vi "Module_p_control_sing_v1.vi"() -> ()   [LabVIEW 2014]
uses:
  <vilib>/rvi/FXPMathLib/FxpAtan2/subVIs/nifxpmath_Atan2_SimConfig.ctl
  <vilib>/rvi/FXPMathLib/FxpSinAndCos/subVIs/nifxpmath_SinAndCos_SimConfig.ctl
  <vilib>/rvi/Emulation/niFpgaGetClockAttributes.vi
  <vilib>/rvi/Emulation/niFpgaSctlEmulationGetInTimedLoop.vi
  <vilib>/rvi/Emulation/niFpgaEmulationReportErrorSimple.vi
  <vilib>/rvi/eio/common/nirviEmuTemplateMethod_errors.vi
  <vilib>/rvi/Emulation/niFpgaProcessEmulError.vi
  <vilib>/rvi/Emulation/niFpgaCriticalErrorInLSC.vi
  <vilib>/rvi/interface/RandomDataEmulation/nirviRandomDataMultiElementFPGAFIFO.vi
  <instcachedir>/0/nirviRandomDataMultiElementFPGAFIFO_AD0CFC12EF974623A9C2E4184BC062B2.lvgen/nirviRandomDataMultiElementFPGAFIFO_AD0CFC12EF974623A9C2E4184BC062B2_023.vi
  <vilib>/rvi/interface/RandomDataEmulation/niFpgaRandomDataHandleErrors.vi
  <vilib>/rvi/FXPMathLib/FxpSinAndCos/simVIs/DllFxpSinAndCosTemp_sub.vi
  <vilib>/rvi/FXPMathLib/FxpAtan2/simVIs/DllFxpAtan2Temp_sub.vi
  <vilib>/eio/EIONode/EIONode.xnode
  <vilib>/rvi/FXPMathLib/FxpMul/XNode/nifxpmath_Multiplier.xnode
  <vilib>/rvi/FXPMathLib/FxpSub/XNode/nifxpmath_Sub.xnode
  <vilib>/rvi/FXPMathLib/FxpAdd/XNode/nifxpmath_Add.xnode
  <vilib>/rvi/Analysis/measure/butterworth/XNode/niFpgaButterworthFilter.xnode
  <vilib>/rvi/DataTransferAndStorage/Container/XNode/niFpgaContainer.xnode
  <vilib>/rvi/interface/RandomDataEmulation/nirviRandomDataFpgaMultiElementTemplate.vi
  <vilib>/rvi/FXPMathLib/FxpSinAndCos/XNode/nifxpmath_SinAndCos.xnode
  <vilib>/rvi/FXPMathLib/FxpAtan2/XNode/nifxpmath_Atan2.xnode
  <vilib>/rvi/FXPMathLib/sim/FxpSim.dll
panel:
  in  "Dy_d_M_avg_Tc (uSec)":u32 caption="M_avg_Tc (uSec)"
  out "Omega_y(rad/s)":fxp<+/-,32,18>
  out "Omega_y(M_avg)":fxp<+/-,32,18>
  out "Omega_y(M)":fxp<+/-,32,18>
  in  "Count(s)":u32
  out "Boolean":bool
  out "Dy_temp":fxp<+/-,22,7>
  in  "Sin ini":bool
  out "Dy_dd":fxp<+/-,25,15>
  in  "scaled coefficients_Dy_dd":i32[](array[numeric])=[1067016412, 3362706]
  in  "Dyr":fxp<+/-,22,8>
  out "Dabr_sin/cos":fxp<+/-,22,8>
  in  "Sin_offset_y":fxp<+/-,12,8>
  in  "Sin_magnitude_y":fxp<+/-,11,8>
  out "Dabr_d":fxp<+/-,33,10>
  out "Sin_omega":fxp<+,29,9>
  out "Dabr_dd":fxp<+/-,34,12>
  in  "Sin wave frenqueny (Hz)":fxp<+,21,5>
  out "Dy_d(M_avg method)":fxp<+/-,32,12>
  in  "Dy_d_M_Tc (mSec)":u32 format="%#_6f"
  out "Dy_d(M method)":fxp<+/-,32,12>
  in  "Method case":i32
  out "Dy_d(T method)":fxp<+/-,32,12>
  in  "mt0_omega":u32
  out "mt_omega":u32
  out "Dy_d(mm/s)":fxp<+/-,32,12>
  out "Sin wave time (s)":fxp<+,64,32>
  in  "Coe Ini":bool
  in  "Encoder Reset_y":bool
  in  "Stop Motor_y":bool
  in  "Kd_y":fxp<+,26,2>
  in  "Kp_y":fxp<+,11,7>=0.375
  out "Dy_error":fxp<+/-,21,11>
  out "Dy_PID":fxp<+/-,21,11>
  in  "Dy_tolerance":fxp<+,32,9>=1.0
  out "Encoder Position_y":i32
  out "rad(NrTheta)_y":fxp<+/-,33,18> format="%.21g"
  out "Dy(mm)":fxp<+/-,22,7>
  out "Omega_y(T)":fxp<+/-,20,9>
  out "vq_y_F":fxp<+/-,20,5> format="%.57g"
  out "vd_y_F":fxp<+/-,20,5>
  out "va_y":fxp<+/-,20,5> format="%.21g"
  out "vb_y":fxp<+/-,20,5> format="%.21g"
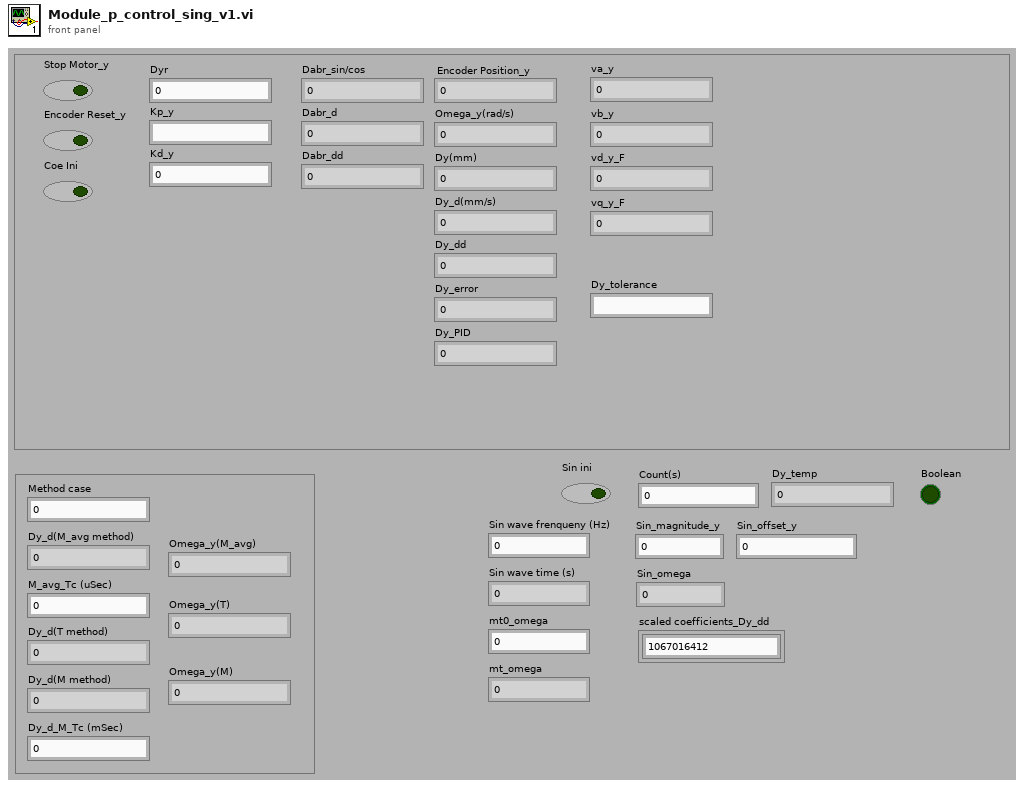
[diagram p1: front panel]
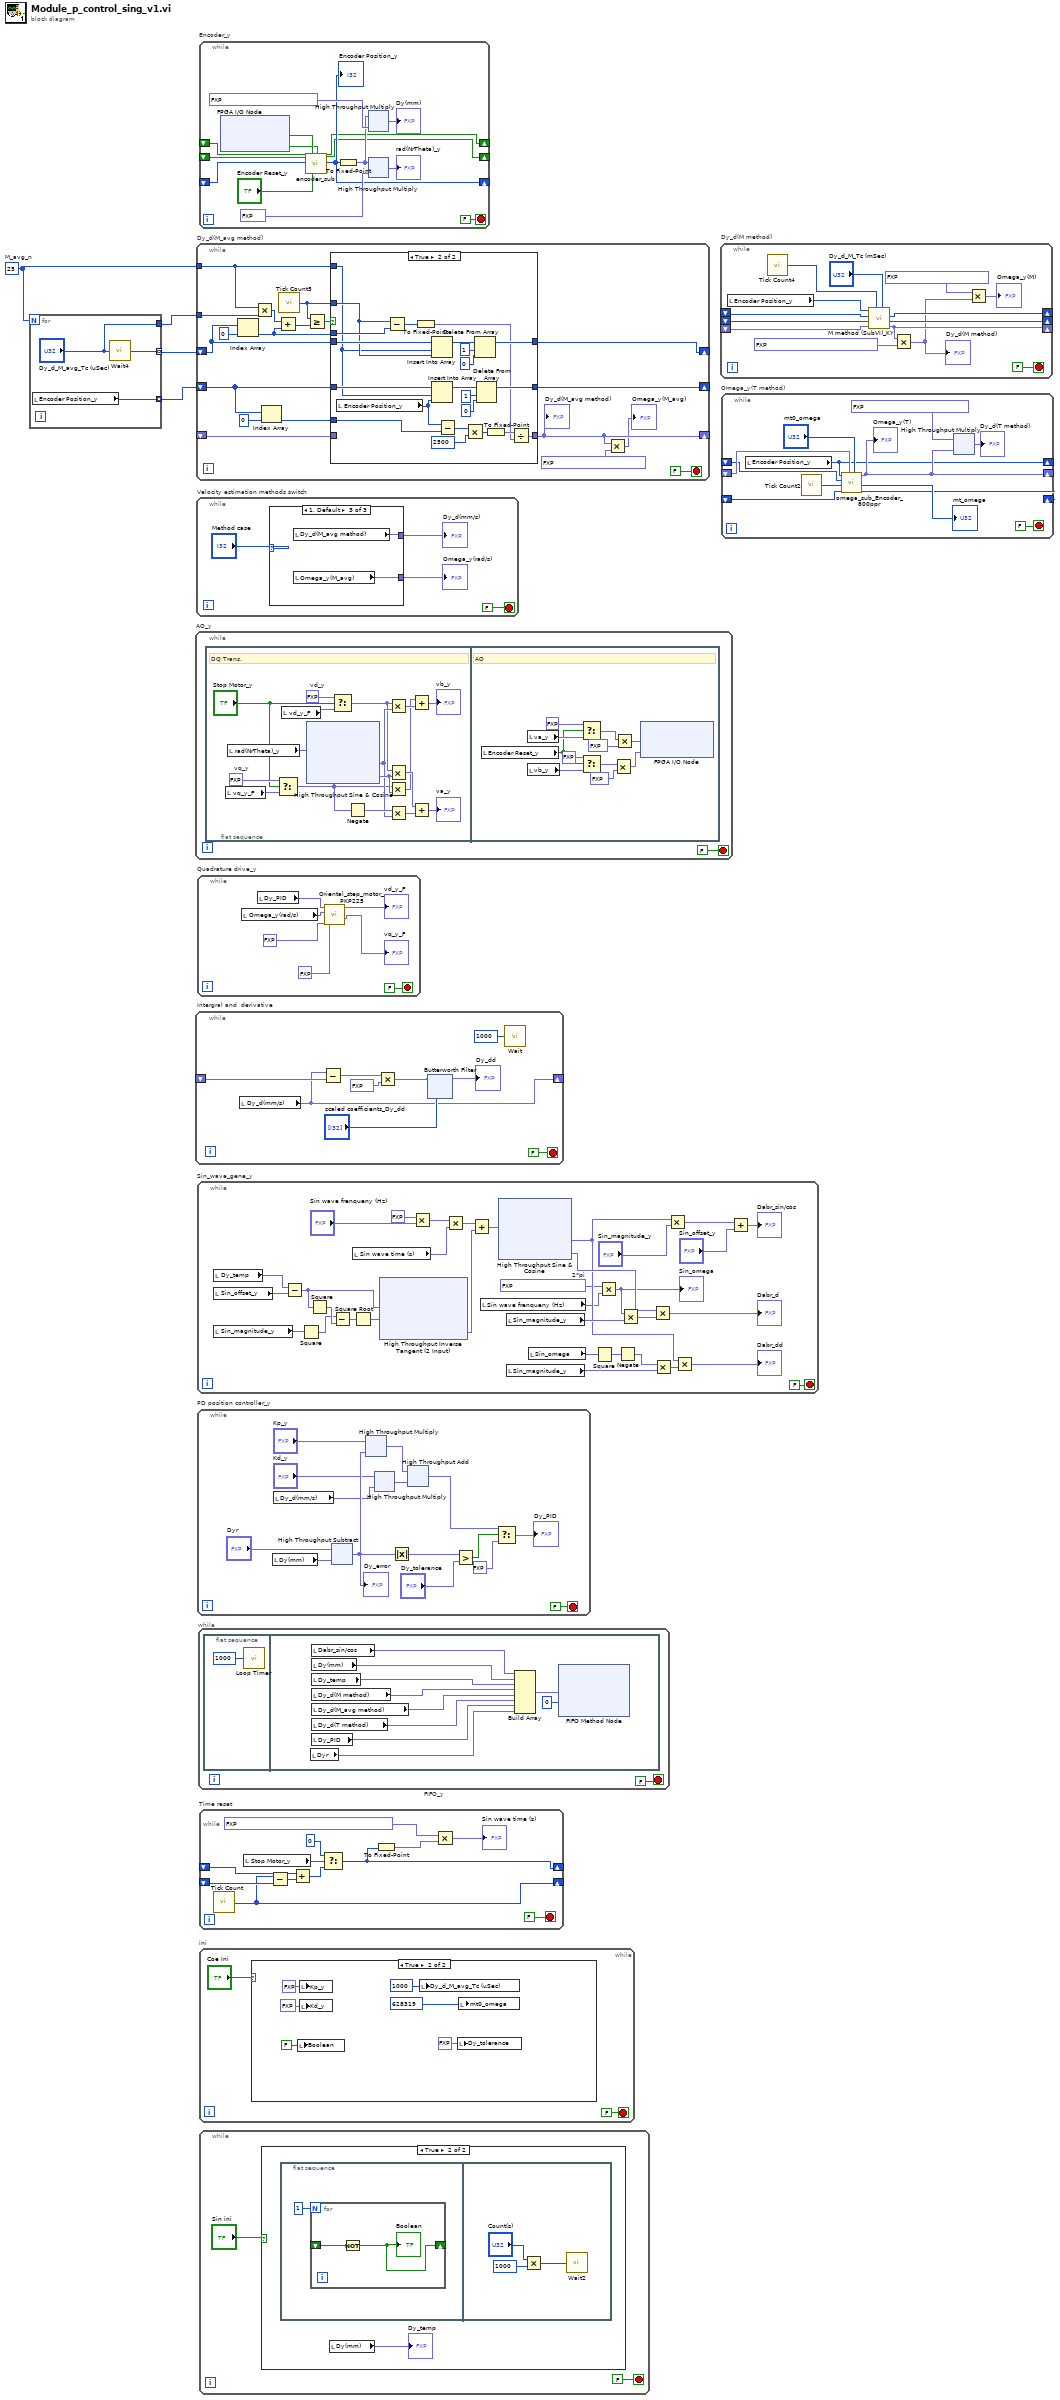
[diagram p0: block diagram]
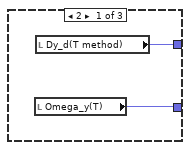
[diagram p4: hidden frame]
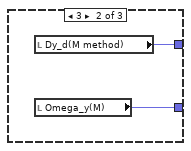
[diagram p5: hidden frame]
diagram:
  w3 = 25  # M_avg_n
  n1 = for {
    N: w3 -> [_]
    tunnel: [w7] -> w1 mode=indexing
    tunnel: [w5] -> w2 mode=indexing
    tunnel: ["Dy_d_M_avg_Tc (uSec)"] -> w4
    n2 = local read "Encoder Position_y"() -> (w5:i32)
    n3 = call "Wait4"("Count(uSec)"="Dy_d_M_avg_Tc (uSec)") -> ("Tick Count(uSec)"=w7:u32)
  }
  n4 = while "AO_y" {
    stop <- FALSE stop-if-true
    n5 = flat-sequence {
      frame #0 {
        w15 = fxp<+/-,20,5> 0.0  # vq_y
        w14 = fxp<+/-,20,5> 0.0  # vd_y
        # "DQ Trans."
        n6 = local read "vq_y_F"() -> (w12:fxp<+/-,20,5>)
        n7 = local read "rad(NrTheta)_y"() -> (w25:fxp<+/-,33,18>)
        n8 = Select(t=w15, s="Stop Motor_y", f=w12) -> (s? t:f=w9:fxp<+/-,20,5>)
        n9 = local read "vd_y_F"() -> (w13:fxp<+/-,20,5>)
        n10 = xnode "High Throughput Sine & Cosine"("x (pi)"=w25) -> ("sin(x)"=w16:fxp<+/-,17,2>, "cos(x)"=w17:fxp<+/-,17,2>)
        n11 = Select(t=w14, s="Stop Motor_y", f=w13) -> (s? t:f=w10:fxp<+/-,20,5>)
        n12 = Negate(x=w9) -> (-x=w24:fxp<+/-,21,6>)
        n13 = Multiply(x=w10, y=w16) -> (x*y=w20:fxp<+/-,20,5>)
        n14 = Multiply(x=w10, y=w17) -> (x*y=w23:fxp<+/-,20,5>)
        n15 = Multiply(x=w9, y=w17) -> (x*y=w19:fxp<+/-,20,5>)
        n16 = Multiply(x=w24, y=w16) -> (x*y=w22:fxp<+/-,20,5>)
        n17 = Add(x=w19, y=w20) -> (x+y=→"vb_y":fxp<+/-,20,5>)
        n18 = Add(x=w23, y=w22) -> (x+y=→"va_y":fxp<+/-,20,5>)
      }
      frame #1 {
        # "AO"
        n19 = local read "Encoder Reset_y"() -> (w62:bool)
        n20 = local read "va_y"() -> (w63:fxp<+/-,20,5>)
        n21 = local read "vb_y"() -> (w64:fxp<+/-,20,5>)
        n22 = Select(t=fxp<+/-,20,5> 3.0 ("Mod2/AO4"), s=w62, f=w63) -> (s? t:f=w60:fxp<+/-,20,5>)
        n23 = Select(t=fxp<+/-,20,5> 0.0 ("Mod2/AO4"), s=w62, f=w64) -> (s? t:f=w57:fxp<+/-,20,5>)
        n24 = Multiply(x=w57, y=fxp<+/-,20,5> -0.5) -> (x*y=w56:fxp<+/-,20,5>)
        n25 = Multiply(x=w60, y=fxp<+/-,20,5> -0.5) -> (x*y=w61:fxp<+/-,20,5>)
        n26 = xnode "FPGA I/O Node"("Mod8/AO0"=w61, "Mod8/AO1"=w56) -> ()  [unwired: 2 in, 2 out]
      }
    }
  }
  n27 = while "Intergral and  derivative" {
    shift-right: [w67] -> _
    shift-left: _ -> [w68]
    stop <- FALSE stop-if-true
    n28 = local read "Dy_d(mm/s)"() -> (w67:fxp<+/-,32,12>)
    n29 = Subtract(x=w67, y=w68) -> (x-y=w70:fxp<+/-,33,13>)
    n30 = Multiply(x=w70, y=fxp<+,10,10> 1000.0) -> (x*y=w71:fxp<+/-,25,15>)
    n31 = xnode "Butterworth Filter"("input data"=w71, "scaled coefficients"="scaled coefficients_Dy_dd") -> ("output data"=→"Dy_dd":fxp<+/-,25,15>)  [unwired: 1 in]
    n32 = call "Wait"("Count(uSec)"=u32 1000 ("Count(mSec)")) -> ()  [unwired: 1 out]
  }
  n33 = while "Dy_d(M_avg method)" {
    shift-right: [w94] -> _
    shift-left: w1 -> [w97]
    tunnel: w3 -> [w95]
    shift-right: [w92] -> _
    shift-left: w2 -> [w90]
    shift-right: [w85] -> _
    shift-left: _ -> [w88]
    tunnel: w4 -> [w87]
    stop <- FALSE stop-if-true
    n34 = Index Array(array=w97, index=0) -> (element=w93:u32)
    n35 = Multiply(x=w95, y=w87) -> (x*y=w100:u32)
    n36 = Index Array(array=w90, index=0) -> (element=w89:i32)
    n37 = Add(x=w100, y=w93) -> (x+y=w99:u32)
    n38 = call "Tick Count5"() -> ("Tick Count(uSec)"=w96:u32)
    n39 = Greater Or Equal?(x=w96, y=w99) -> (x >= y?=w98:bool)
    n40 = case shown="True" w98 {
      tunnel: w97 -> [w105 w127]
      tunnel: w96 -> [_ w121]
      tunnel: w95 -> [_ w110]
      tunnel: [w105 w123] -> w94
      tunnel: w93 -> [_ w122]
      tunnel: w90 -> [w104 w111]
      tunnel: [w104 w109] -> w92
      tunnel: [w103 w108] -> w85
      tunnel: w89 -> [_ w106]
      tunnel: w88 -> [w103 _]
      frame False {
      }
      frame True {
        n41 = local read "Encoder Position_y"() -> (w115:i32)
        n42 = Subtract(x=w121, y=w122) -> (x-y=w120:u32)
        n43 = To Fixed-Point(number=w120) -> (fixed-point=w107:fxp<+,32,32>)  [unwired: 1 in]
        n44 = Insert Into Array(array=w127, index=w110, new element=w121) -> (w126:u32[])
        n45 = Insert Into Array(array=w111, index=w110, new element=w115) -> (w112:i32[])
        n46 = Subtract(x=w115, y=w106) -> (x-y=w116:i32)
        n47 = Multiply(x=w116, y=2500) -> (x*y=w118:i32)
        n48 = Delete From Array(array=w126, length=1, index=0) -> (array with subset deleted=w123:u32[])  [unwired: 1 out]
        n49 = Delete From Array(array=w112, length=1, index=0) -> (array with subset deleted=w109:i32[])  [unwired: 1 out]
        n50 = To Fixed-Point(number=w118) -> (fixed-point=w119:fxp<+/-,32,32>)  [unwired: 1 in]
        n51 = Divide(x=w119, y=w107) -> (x/y=w108:fxp<+/-,32,12>)
      }
    }
    "Dy_d(M_avg method)" <- w85
    n52 = Multiply(x=w85, y=fxp<+/-,32,12> 3.1415929794311523 ("x")) -> (x*y=→"Omega_y(M_avg)":fxp<+/-,32,18>)
  }
  n53 = while "Velocity estimation methods switch" {
    stop <- FALSE stop-if-true
    n54 = case shown="1, Default" "Method case" {
      tunnel: [w132 w134 w136] -> w129
      tunnel: [w133 w135 w137] -> w128
      frame 2 {
        n55 = local read "Omega_y(T)"() -> (w133:fxp<+/-,20,9>)
        n56 = local read "Dy_d(T method)"() -> (w132:fxp<+/-,32,12>)
      }
      frame 3 {
        n57 = local read "Dy_d(M method)"() -> (w134:fxp<+/-,32,12>)
        n58 = local read "Omega_y(M)"() -> (w135:fxp<+/-,32,18>)
      }
      frame 1, Default {
        n59 = local read "Dy_d(M_avg method)"() -> (w136:fxp<+/-,32,12>)
        n60 = local read "Omega_y(M_avg)"() -> (w137:fxp<+/-,32,18>)
      }
    }
    "Dy_d(mm/s)" <- w129
    "Omega_y(rad/s)" <- w128
  }
  n61 = while "Quadrature drive_y" {
    stop <- FALSE stop-if-true
    n62 = local read "Omega_y(rad/s)"() -> (w140:fxp<+/-,32,18>)
    n63 = local read "Dy_PID"() -> (w141:fxp<+/-,21,11>)
    n64 = call "Oriental_step_motor_PKP225.vi"("F_Threshold"=fxp<+,12,12> 10.0, "dFmr"=fxp<+/-,25,15> 0.0 ("f"), "omega"=w140, "Fmr"=w141) -> ("vq_F"=→"vq_y_F":fxp<+/-,20,5>, "vd_F"=→"vd_y_F":fxp<+/-,20,5>)  [unwired: 6 in]
  }
  n65 = while "Sin_wave_gene_y" {
    stop <- FALSE stop-if-true
    w150 = fxp<+,20,3> 6.2831878662109375  # 2*pi
    n66 = local read "Dy_temp"() -> (w172:fxp<+/-,22,7>)
    n67 = local read "Sin_offset_y"() -> (w171:fxp<+/-,12,8>)
    n68 = local read "Sin_magnitude_y"() -> (w170:fxp<+/-,11,8>)
    n69 = Subtract(x=w172, y=w171) -> (x-y=w169:fxp<+/-,24,9>)
    n70 = Square(x=w170) -> (x^2=w167:fxp<+,21,15>)
    n71 = Square(x=w169) -> (x^2=w168:fxp<+,46,16>)
    n72 = Subtract(x=w167, y=w168) -> (x-y=w166:fxp<+,47,17>)
    n73 = local read "Sin wave time (s)"() -> (w152:fxp<+,64,32>)
    n74 = Square Root(x=w166) -> (sqrt(x)=w165:fxp<+,50,9>)
    n75 = xnode "High Throughput Inverse Tangent (2 Input)"("y"=w169, "x"=w165) -> ("atan2(y,x) (pi)"=w173:fxp<+/-,16,2>)
    n76 = Multiply(x=fxp<+,1,2> 2.0 ("y"), y="Sin wave frenqueny (Hz)") -> (x*y=w153:fxp<+,21,6>)
    n77 = Multiply(x=w153, y=w152) -> (x*y=w151:fxp<+,48,18>)
    n78 = Add(x=w151, y=w173) -> (x+y=w174:fxp<+/-,50,20>)
    n79 = local read "Sin wave frenqueny (Hz)"() -> (w148:fxp<+,21,5>)
    n80 = xnode "High Throughput Sine & Cosine"("x (pi)"=w174) -> ("sin(x)"=w156:fxp<+/-,17,2>, "cos(x)"=w162:fxp<+/-,17,2>)
    n81 = local read "Sin_magnitude_y"() -> (w164:fxp<+/-,11,8>)
    n82 = local read "Sin_magnitude_y"() -> (w161:fxp<+/-,11,8>)
    n83 = local read "Sin_omega"() -> (w160:fxp<+,29,9>)
    n84 = Square(x=w160) -> (x^2=w159:fxp<+,35,15>)
    n85 = Multiply(x=w150, y=w148) -> (x*y=w149:fxp<+,29,9>)
    "Sin_omega" <- w149
    n86 = Negate(x=w159) -> (-x=w158:fxp<+/-,36,16>)
    n87 = Multiply(x=w149, y=w164) -> (x*y=w163:fxp<+,31,9>)
    n88 = Multiply(x=w162, y=w163) -> (x*y=→"Dabr_d":fxp<+/-,33,10>)
    n89 = Multiply(x=w158, y=w161) -> (x*y=w157:fxp<+/-,34,12>)
    n90 = Multiply(x=w156, y="Sin_magnitude_y") -> (x*y=w177:fxp<+/-,20,8>)
    n91 = Multiply(x=w156, y=w157) -> (x*y=→"Dabr_dd":fxp<+/-,34,12>)
    n92 = Add(x=w177, y="Sin_offset_y") -> (x+y=→"Dabr_sin/cos":fxp<+/-,22,8>)
  }
  n93 = while "PD position controller_y" {
    stop <- FALSE stop-if-true
    n94 = local read "Dy(mm)"() -> (w245:fxp<+/-,22,7>)
    n95 = local read "Dy_d(mm/s)"() -> (w241:fxp<+/-,32,12>)
    n96 = xnode "High Throughput Subtract"("x"="Dyr", "y"=w245) -> ("x-y"=w247:fxp<+/-,24,9>)
    "Dy_error" <- w247
    n97 = xnode ("High Throughput Multiply")("x"="Kp_y", "y"=w247) -> ("x*y"=w246:fxp<+/-,33,17>)
    n98 = xnode ("High Throughput Multiply")("x"="Kd_y", "y"=w241) -> ("x*y"=w244:fxp<+/-,31,21>)
    n99 = Absolute Value(x=w247) -> (abs(x)=w249:fxp<+,24,9>)
    n100 = xnode ("High Throughput Add")("x"=w246, "y"=w244) -> ("x+y"=w237:fxp<+/-,21,11>)
    n101 = Greater?(x=w249, y="Dy_tolerance") -> (0:w248:bool)
    n102 = Select(t=w237, s=w248, f=fxp<+/-,21,11> 0.0) -> (s? t:f=→"Dy_PID":fxp<+/-,21,11>)
  }
  n103 = while "FIFO_y" {
    stop <- FALSE stop-if-true
    n104 = flat-sequence {
      frame #0 {
        n105 = call "Loop Timer"("Count(uSec)"=u32 1000 ("Loop Period (usec)")) -> ()  [unwired: 1 out]
      }
      frame #1 {
        n106 = local read "Dyr"() -> (w262:fxp<+/-,22,8>)
        n107 = local read "Dabr_sin/cos"() -> (w259:fxp<+/-,22,8>)
        n108 = local read "Dy(mm)"() -> (w258:fxp<+/-,22,7>)
        n109 = local read "Dy_temp"() -> (w257:fxp<+/-,22,7>)
        n110 = local read "Dy_d(M method)"() -> (w263:fxp<+/-,32,12>)
        n111 = local read "Dy_d(M_avg method)"() -> (w256:fxp<+/-,32,12>)
        n112 = local read "Dy_d(T method)"() -> (w254:fxp<+/-,32,12>)
        n113 = local read "Dy_PID"() -> (w255:fxp<+/-,21,11>)
        n114 = Build Array(w259, w258, w257, w263, w256, w254, w255, w262) -> (w260:fxp<+/-,32,12>[])
        n115 = xnode ("FIFO Method Node")("Element"=w260, "Timeout"=0) -> ()  [unwired: 1 in, 2 out]
      }
    }
  }
  n116 = while "Encoder_y" {
    shift-right: [w265] -> _
    shift-left: _ -> [w277]
    shift-right: [w264] -> _
    shift-left: _ -> [w276]
    shift-right: [w269] -> _
    shift-left: _ -> [w275]
    stop <- FALSE stop-if-true
    n117 = xnode "FPGA I/O Node"() -> ("Mod4/DI3"=w267:bool, "Mod4/DI4"=w266:bool)  [unwired: 2 in, 2 out]
    n118 = call "encoder_sub.vi"("A_pre"=w277, "B_pre"=w276, "Encoder Position_pre"=w275, "A input"=w267, "Encoder Position Reset"="Encoder Reset_y", "B input"=w266) -> ("A"=w265:bool, "B"=w264:bool, "Encoder Position (Counts)"=w269:i32)  [unwired: 19 in]
    "Encoder Position_y" <- w269
    n119 = To Fixed-Point(number=w269) -> (fixed-point=w272:fxp<+/-,18,18>)  [unwired: 1 in]
    n120 = xnode ("High Throughput Multiply")("x"=w272, "y"=fxp<+/-,15,-7> 0.0025000572204589844) -> ("x*y"=→"Dy(mm)":fxp<+/-,22,7>)
    n121 = xnode ("High Throughput Multiply")("x"=w272, "y"=fxp<+,24,0> 0.125) -> ("x*y"=→"rad(NrTheta)_y":fxp<+/-,33,18>)
  }
  n122 = while "Time reset" {
    shift-right: [w289] -> _
    shift-left: _ -> [w290]
    shift-right: [w281] -> _
    shift-left: _ -> [w283]
    stop <- FALSE stop-if-true
    n123 = call "Tick Count"() -> ("Tick Count(uSec)"=w289:u32)
    n124 = local read "Stop Motor_y"() -> (w286:bool)
    n125 = Subtract(x=w289, y=w290) -> (x-y=w285:u32)
    n126 = Add(x=w283, y=w285) -> (x+y=w284:u32)
    n127 = Select(t=u32 0, s=w286, f=w284) -> (s? t:f=w281:u32)
    n128 = To Fixed-Point(number=w281) -> (fixed-point=w279:fxp<+,64,32>)  [unwired: 1 in]
    n129 = Multiply(x=fxp<+,20,-18> 1.0000003385357559e-06 ("y"), y=w279) -> (x*y=→"Sin wave time (s)":fxp<+,64,32>)
  }
  n130 = while "ini" {
    stop <- FALSE stop-if-true
    n131 = case shown="True" "Coe Ini" {
      frame False {
      }
      frame True {
        n132 = local write "Boolean"(FALSE ("dF_PID_add")) -> ()
        n133 = local write "Kp_y"(fxp<+,11,7> 40.0 ("Kpb")) -> ()
        n134 = local write "Kd_y"(fxp<+,26,2> 0.5 ("Kdb")) -> ()
        n135 = local write "Dy_d_M_avg_Tc (uSec)"(u32 1000 ("M_avg_Tc (uSec)")) -> ()
        n136 = local write "Dy_tolerance"(fxp<+,32,9> 1.0 ("Dy_tolerance")) -> ()
        n137 = local write "mt0_omega"(u32 628319 ("mt0_omega")) -> ()
      }
    }
  }
  n138 = while {
    stop <- FALSE stop-if-true
    n139 = case shown="True" "Sin ini" {
      frame False {
      }
      frame True {
        n140 = flat-sequence {
          frame #0 {
            n141 = for {
              N: 1 -> [_]
              shift-right: [w303] -> _
              shift-left: _ -> [w304]
              n142 = Not(x=w304) -> (.not. x?=w303:bool)
              "Boolean" <- w303
            }
          }
          frame #1 {
            n143 = Multiply(x="Count(s)", y=u32 1000) -> (x*y=w305:u32)
            n144 = call "Wait2"("Count(mSec)"=w305) -> ()  [unwired: 1 out]
          }
        }
        n145 = local read "Dy(mm)"() -> (→"Dy_temp":fxp<+/-,22,7>)
      }
    }
  }
  n146 = while "Dy_d(M method)" {
    shift-right: [w319] -> _
    shift-left: _ -> [w314]
    shift-right: [w318] -> _
    shift-left: _ -> [w313]
    shift-right: [w311] -> _
    shift-left: _ -> [w312]
    stop <- FALSE stop-if-true
    n147 = local read "Encoder Position_y"() -> (w315:i32)
    n148 = call "Tick Count4"() -> ("Tick Count(mSec)"=w316:u32)
    n149 = call "M method (SubVI)_KY.vi"("Tc (mSec)"="Dy_d_M_Tc (mSec)", "Tick Count (mSec)"=w316, "Encoder velocity_pre (pulse/s)"=w312, "Shift Register in 2"=w313, "Shift Register in 1"=w314, "Encoder pulses"=w315) -> ("Encoder velocity (pulse/s)"=w311:fxp<+/-,64,32>, "Shift Register out 2"=w318:i32, "Shift Register out 1"=w319:u32)  [unwired: 3 in]
    n150 = Multiply(x=w311, y=fxp<+/-,20,-5> 0.002499997615814209) -> (x*y=w310:fxp<+/-,32,12>)
    "Dy_d(M method)" <- w310
    n151 = Multiply(x=fxp<+/-,32,12> 3.1415929794311523, y=w310) -> (x*y=→"Omega_y(M)":fxp<+/-,32,18>)
  }
  n152 = while "Omega_y(T method)" {
    shift-right: [w324] -> _
    shift-left: _ -> [w323]
    shift-right: [w322] -> _
    shift-left: _ -> [w329]
    shift-right: [w327] -> _
    shift-left: _ -> [w325]
    stop <- FALSE stop-if-true
    n153 = local read "Encoder Position_y"() -> (w324:i32)
    n154 = call "Tick Count2"() -> ("Tick Count(Ticks)"=w330:u32)
    n155 = call "omega_sub_Encoder_800ppr.vi"("mt0"="mt0_omega", "omega_pre"=w325, "ticks_m_pre"=w329, "ticks"=w330, "count_pre"=w323, "count"=w324) -> ("ticks_m"=w322:u32, "mt"=→"mt_omega":u32, "omega"=w327:fxp<+/-,20,9>)  [unwired: 3 in]
    "Omega_y(T)" <- w327
    n156 = xnode ("High Throughput Multiply")("x"=fxp<+/-,26,1> 0.3183099031448364, "y"=w327) -> ("x*y"=→"Dy_d(T method)":fxp<+/-,32,12>)
  }
